vi "FGV_FromUserMEssageEvent.vi"(7 "Command":T1, 8 "error in":errorcluster) -> (0 "error out":errorcluster, 3 "FromUserMessageEvent":refnum<user-event>)   [LabVIEW 2013]
uses:
  EnumFgvEventCommand.ctl
  FromUserMessageEvent.ctl
  FromUserMessageEvent_Orders.ctl
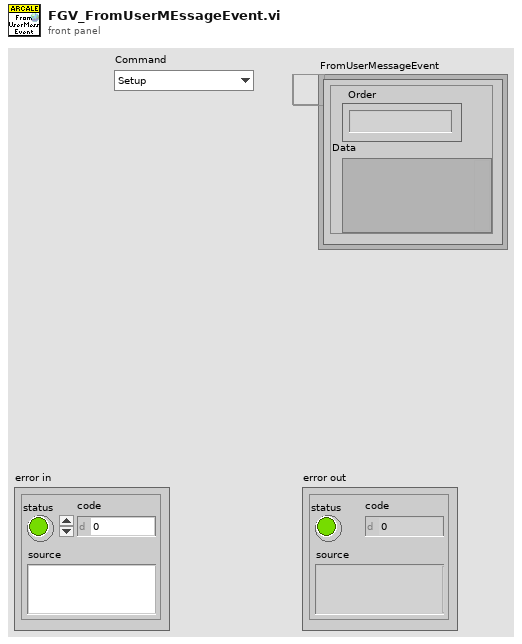
[diagram p1: front panel]
types:
  T1 = typedef "EnumFgvEventCommand.ctl" = enum16{"Setup", "Cleanup", "Get"}
  T2 = typedef "FromUserMessageEvent.ctl" = cluster{"Order":T3, "Data":variant}
  T3 = typedef "FromUserMessageEvent_Orders.ctl" = enum16{"Wait for user action", "NaO", "PM finished executing", "Update UUT Test Progress", "Update Test Seq Names", "Update Test Sequence Result", "Scripter Starts", "Scripter Ended", "UUT Start", "DB Log Starts", "DB Log Ends", "MES UUT Check Starts", "MES UUT Check Ends", "MES UUT Status Starts", "MES UUT Status Ends", "MES UUT Results Starts", "MES UUT Results Ends", "Opening Instruments Ref", "End Opening Instrument Ref", "Update Spec Sequence Name", "Test Failed"}
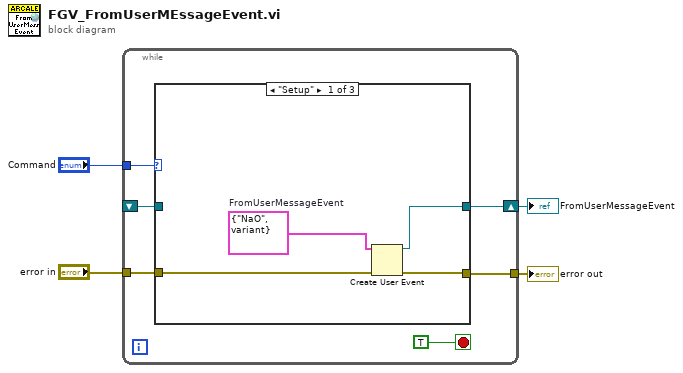
[diagram p0: block diagram]
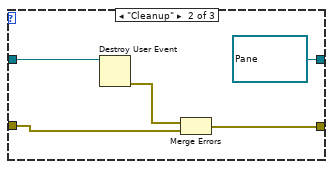
[diagram p2: hidden frame]
diagram:
  n1 = while {
    tunnel: "error in" -> [w8]
    tunnel: "Command" -> [w9]
    tunnel: [w7] -> w2
    shift-right: [w5] -> w1
    shift-left: _ -> [w6]
    stop <- TRUE stop-if-true
    n2 = case shown="\"Setup\"" w9 {
      tunnel: w8 -> [w14 w18 w21]
      tunnel: [w13 w16 w21] -> w7
      tunnel: w6 -> [_ w19 w20]
      tunnel: [w11 refnum<user-event> refnum ("FromUserMessageEvent") w20] -> w5
      frame "Setup" {
        w12 = T2 {"Order"=enum."NaO", "Data"=variant}  # FromUserMessageEvent
        n3 = Create User Event(user event datatype=w12, error in=w14) -> (user event=w11:refnum<user-event>, error out=w13:errorcluster)
      }
      frame "Cleanup" {
        n4 = Destroy User Event(user event=w19) -> (error out=w17:errorcluster)  [unwired: 1 in]
        n5 = Merge Errors(w17, w18) -> (w16:errorcluster)
      }
      frame "Get" {
      }
    }
  }
  "error out" <- w2
  "FromUserMessageEvent" <- w1
